vi "Read Startup.vi"(8 "error in (no error)":errorcluster, 11 "Path (*.ini)":path) -> (0 "error out":errorcluster, 3 "Name,Path":string[][](array[string]))   [LabVIEW 2018, in "Shared.lvlib"]
uses:
  Shared.lvlib
  <vilib>/Utility/config.llb/NI_LVConfig.lvlib
  <vilib>/Utility/config.llb/Read Key (String).vi
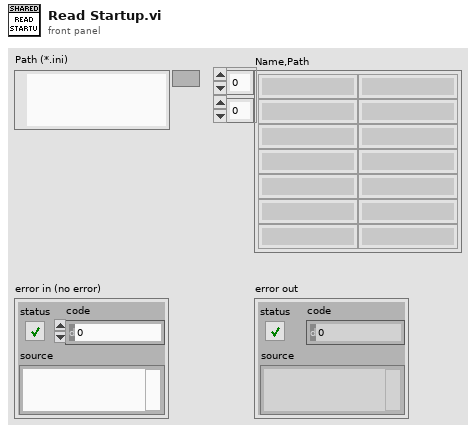
[diagram p1: front panel]
types:
  T1 = typedef "NI_LVConfig.lvlib/Config Data RefNum.ctl" = refnum<k1>
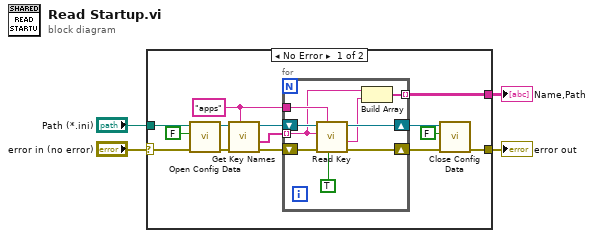
[diagram p0: block diagram]
diagram:
  n1 = case shown="No Error" "error in (no error)" {
    selector: "error in (no error)" -> [w8 w28]
    tunnel: "Path (*.ini)" -> [w7 _]
    tunnel: [w6 w28] -> w2
    tunnel: [w5 _] -> w1
    frame No Error {
      w12 = "apps" ("section")
      n2 = call <vilib>:"Open Config Data.vi"("error in (no error)"=w8, "create file if necessary (T)"=FALSE, "configuration file path"=w7) -> ("error out"=w18:errorcluster, "refnum"=w15:T1)  [unwired: 6 in, 1 out]
      n3 = call <vilib>:"Get Key Names.vi"("section"=w12, "error in (no error)"=w18, "refnum"=w15) -> ("error out"=w16:errorcluster, "key names"=w11:string[], "refnum out"=w13:T1)  [unwired: 5 in, 1 out]
      n4 = for {
        shift-right: [w26] -> w14
        shift-left: w16 -> [w27]
        shift-right: [w23] -> w10
        shift-left: w13 -> [w25]
        tunnel: w12 -> [w22]
        tunnel: w11 -> [w21] mode=indexing
        tunnel: [w20] -> w5 mode=indexing
        n5 = call-poly <vilib>:"Read Key.vi"("read raw string? (F)"=TRUE, "section"=w22, "error in (no error)"=w27, "key"=w21, "refnum"=w25) -> ("error out"=w26:errorcluster, "value"=w19:string, "refnum out"=w23:T1)  [unwired: 3 in, 1 out]
        n6 = Build Array(w21, w19) -> (w20:string[])
      }
      n7 = call <vilib>:"Close Config Data.vi"("error in (no error)"=w14, "write file if changed (T)"=FALSE, "refnum"=w10) -> ("error out"=w6:errorcluster)  [unwired: 7 in, 1 out]
    }
    frame Error {
    }
  }
  "error out" <- w2
  "Name,Path" <- w1
